vi "lisa_functional.vi"() -> ()   [LabVIEW 2019]
doc: "The classic \"Hello World\" example."
uses:
  <vilib>/Enthought/Python Integration Toolkit/api/Console Visibility.ctl
  <vilib>/Analysis/Matrix/Datatypes/ComplexMatrix.ctl
  <vilib>/Enthought/Python Integration Toolkit/api/Unpack String.vi
  <vilib>/Enthought/Python Integration Toolkit/Python Integration Toolkit.lvlib
  <vilib>/Analysis/Matrix/NI_Matrix.lvlib
panel:
  in  "Mode Coefficients (Cnm)":T1
  in  "beam params. 4":cdb
  in  "b(t) 2":dbl
  in  "Scattering Matrix 2":T1
  in  "Static offsets 2":dbl
  in  "Magnification 2":dbl
  in  "a(t) 2":dbl
  in  "Arm Length 2-3 [m]":dbl
  in  "Arm Length 1-3 [m]":dbl
  in  "b(t)5":dbl
  in  "Scattering Matrix 6":T1
  in  "Static offsets 6":dbl
  in  "Magnification 6":dbl
  in  "a(t)5":dbl
  in  "Arm Length 1-2 [m]":dbl
  in  "b(t)5":dbl
  in  "Scattering Matrix 5":T1
  in  "Static offsets 5":dbl
  in  "Magnification 5":dbl
  in  "a(t)5":dbl
  in  "b(t) 4":dbl
  in  "Scattering Matrix 4":T1
  in  "Static offsets 4":dbl
  in  "Magnification 4":dbl
  in  "a(t) 4":dbl
  in  "C n,m 3":T1
  in  "beam params. 3":cdb
  in  "C n,m 2":T1
  in  "beam params. 2":cdb
  in  "b(t) 3":dbl
  in  "Scattering Matrix 3":T1
  in  "Static offsets 3":dbl
  in  "Magnification 3":dbl
  in  "a(t) 3":dbl
  in  "b(t)":dbl
  in  "Scattering Matrix":T1
  in  "Static offsets":dbl
  in  "Magnification":dbl
  in  "a(t)":dbl
  in  "Mode Coefficients (Cnm)":T1
  in  "beam params.":cdb
  in  "Display Python console?":T2=enum."Hide Console"
  in  "Your name":string="LabVIEW Champion"
  out "Response from Python":string
  # "LISA Optical Metrology Functional Panel"
  # "S/C 1"
  # "S/C 3"
  # "MOSA 3(a)"
  # "MOSA 1(a)"
  # "TM 1(a)"
  # "MOSA 1(b)"
  # "Dynamic\nAng. Offsets"
  # "Dynamic\nAng. Offsets"
  # "TM 1(b)"
  # "MOSA 3(b)"
  # "TM 3(a)"
  # "TM 3(b)"
  # "Laser 1(a)"
  # "Backlink"
  # "Dynamic\nAng. Offsets"
  # "Laser 3"
  # "Dynamic\nAng. Offsets"
  # "TS 1(a)"
  # "TS 1(b)"
  # "TS 3(b)"
  # "PD 1(b)"
  # "PD 1(a)"
  # "TM PD\n1(a)"
  # "OB 1(a)"
  # "PRDS"
  # "OB 1(b)"
  # "TS 3(a)"
  # "PRDS"
  # "TM Im\n1(a)"
  # "Ref Im\n1(a)"
  # "Imaging 1(b)"
  # "Imaging 1(a)"
  # "Laser 1(b)"
  # "RX CLIP 1(b)"
  # "RX CLIP 1(a)"
  # "OB 3(a)"
  # "OB 3(b)"
  # "TX CLIP"
  # "RX CLIP"
  # "TX CLIP 1(a)"
  # "PM(tx/rx) 1(b)"
  # "PM(tx/rx) 1(a)"
  # "TX CLIP 1(b)"
  # "S/C 2"
  # "TM 2(a)"
  # "MOSA 2(a)"
  # "MOSA 2(b)"
  # "TS 2(a)"
  # "TM 2(b)"
  # "Dynamic\nAng. Offsets"
  # "Dynamic\nAng. Offsets"
  # "TS 2(b)"
  # "Laser 2"
  # "OB 2(a)"
  # "OB 2(a)"
  # "TX CLIP"
  # "TX CLIP"
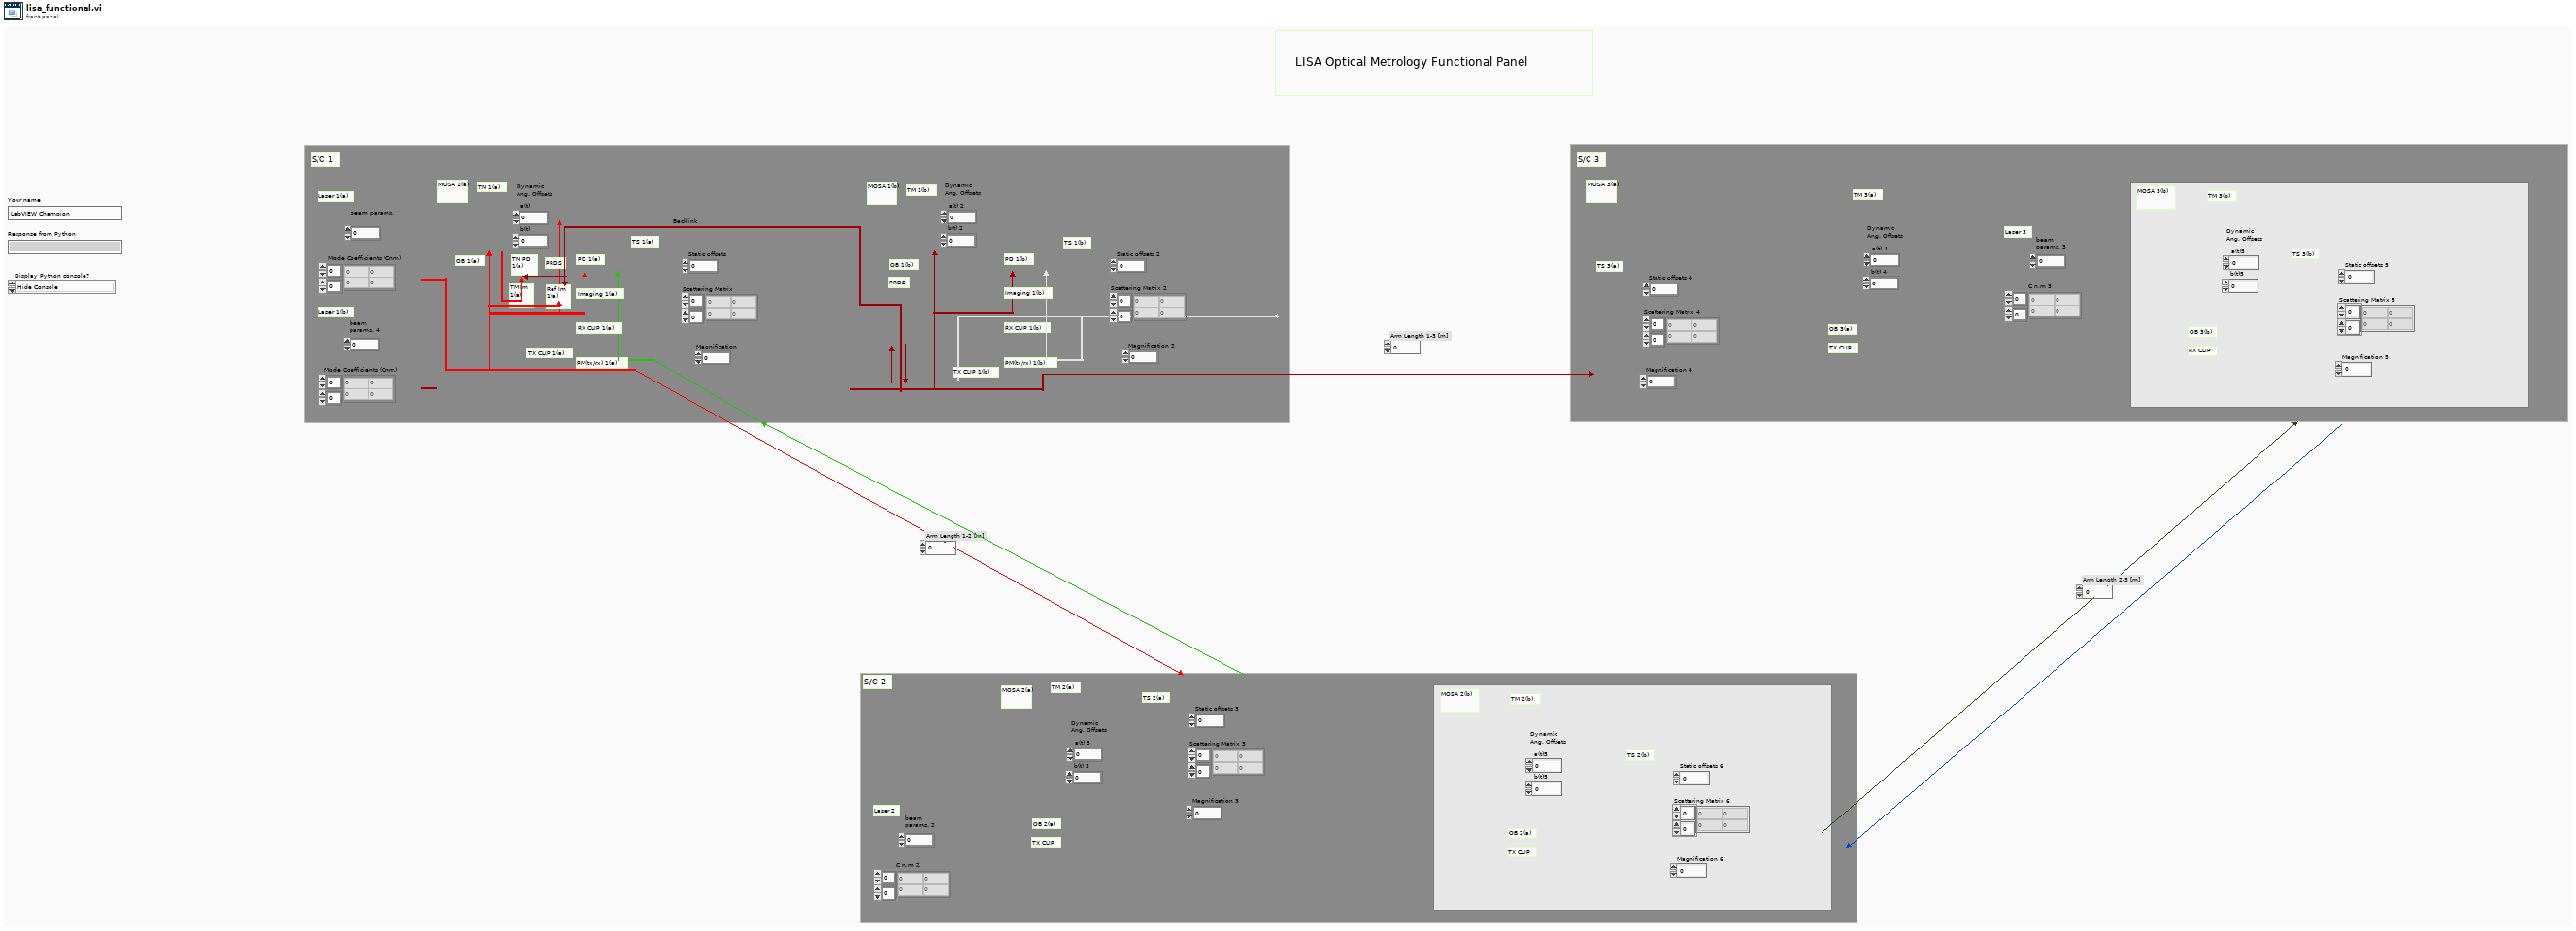
[diagram p1: front panel]
types:
  T1 = typedef "NI_Matrix.lvlib/ComplexMatrix.ctl" = cdb[][]
  T2 = typedef "Python Integration Toolkit.lvlib/Console Visibility.ctl" = enum16{"Show Console", "Show Console While Running", "Hide Console"}
  T3 = typedef "Python Integration Toolkit.lvlib/Session ID.ctl" = u64
  T4 = typedef "Python Integration Toolkit.lvlib/Python Objects.ctl" = variant
  T5 = cluster{"beam params.":cdb, "Mode Coefficients (Cnm)":T1}
  T6 = cluster{cluster{"beam params.":cdb, "Mode Coefficients (Cnm)":T1}, "Scattering Matrix":T1}
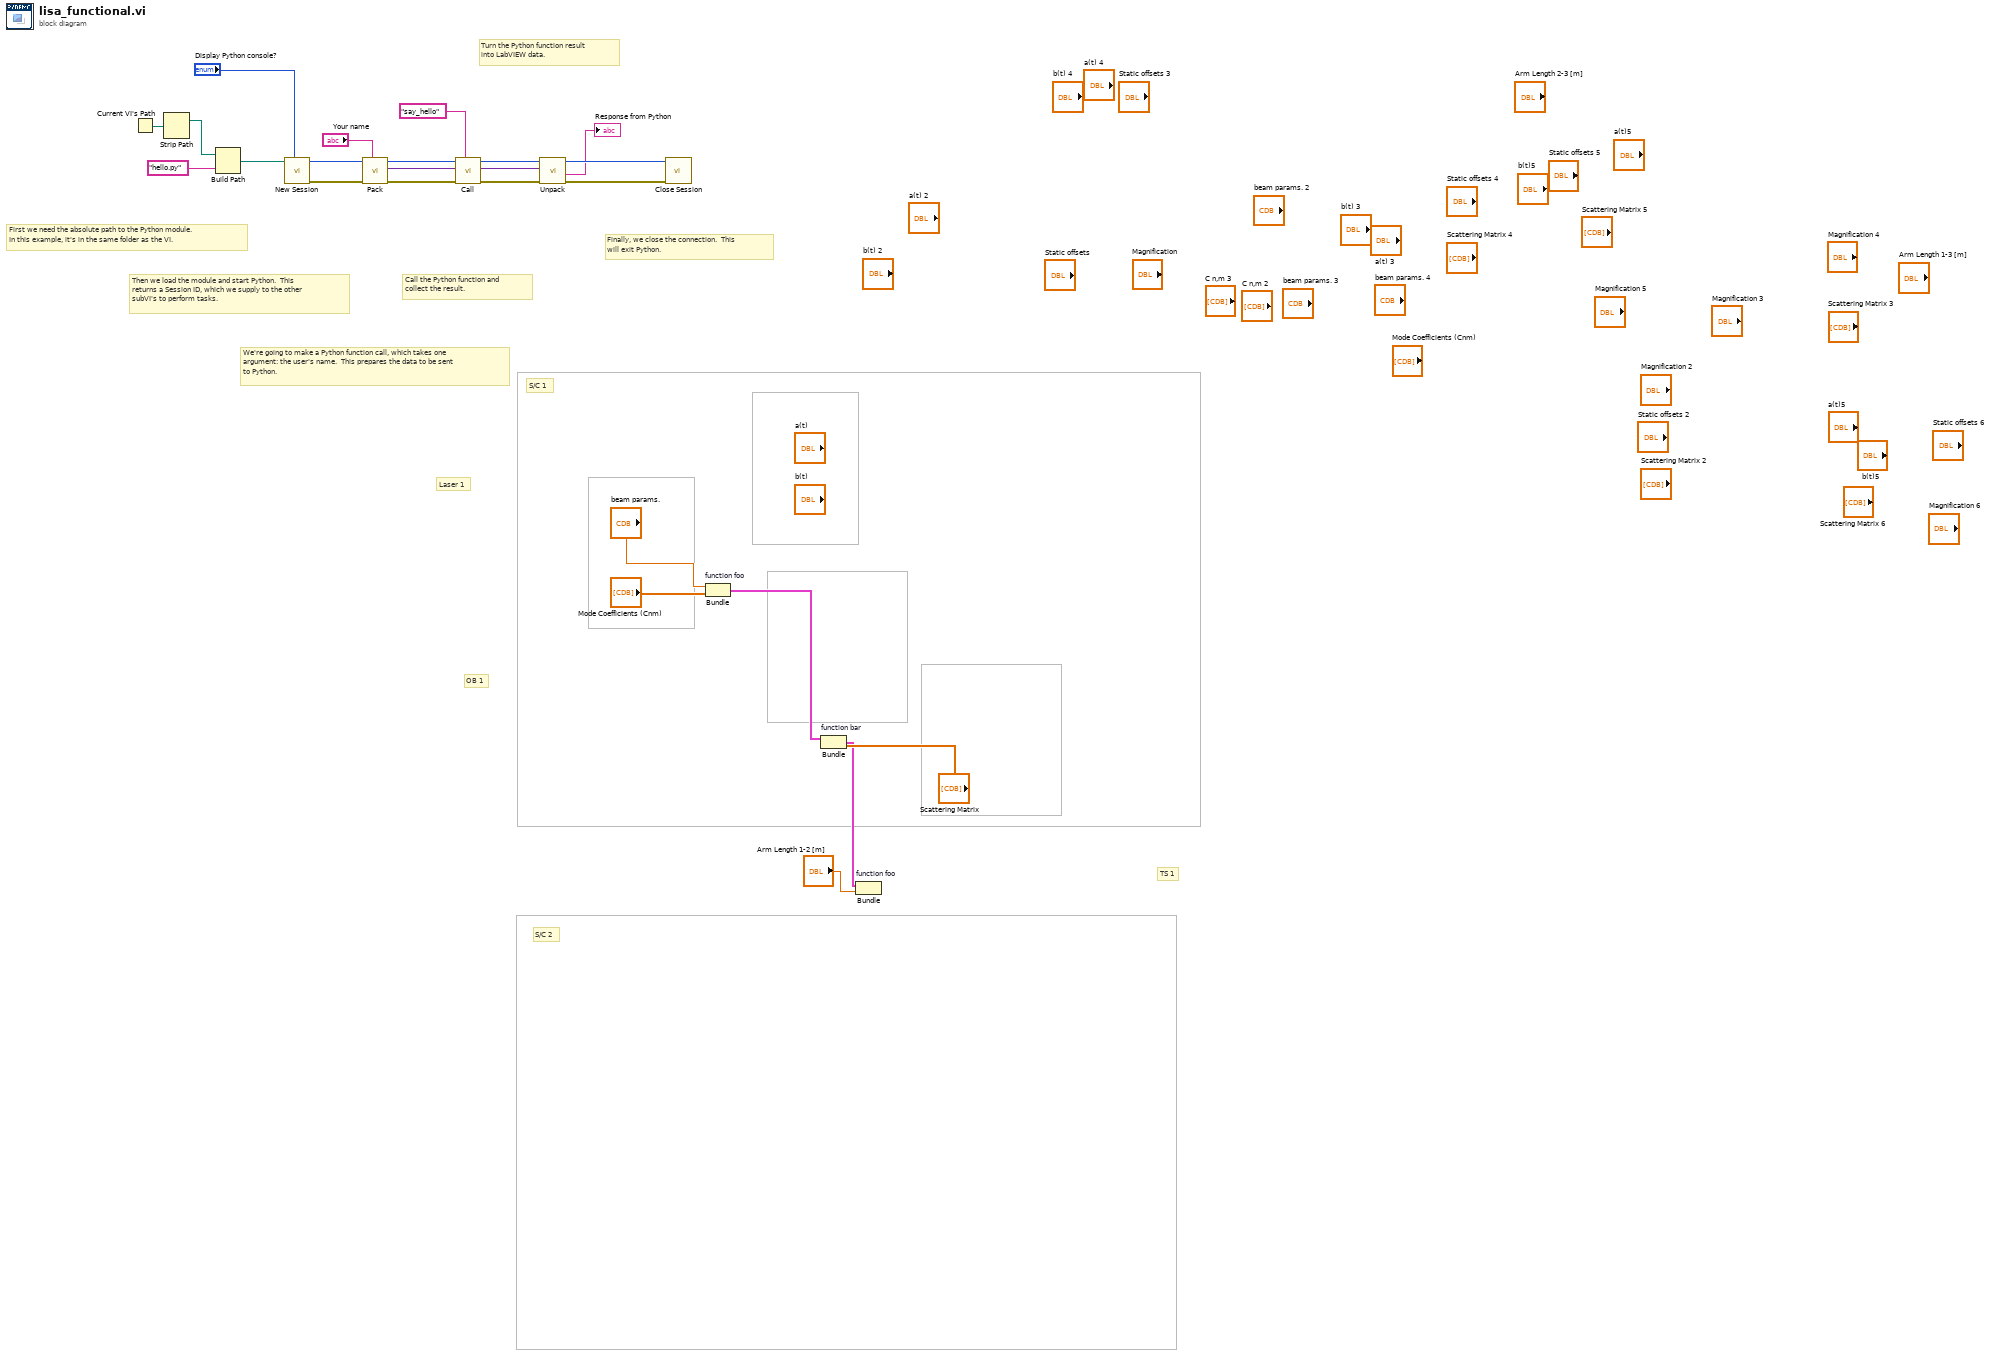
[diagram p0: block diagram]
diagram:
  # "TS 1"
  # "S/C 2"
  # "OB 1"
  # "S/C 1"
  # "Laser 1"
  # "Finally, we close the connection.  This\nwill exit Python."
  # "Turn the Python function result\ninto LabVIEW data."
  # "Call the Python function and\ncollect the result."
  # "We're going to make a Python function call, which takes one\nargument: the user's name.  This prepares the data to be sent\nto Python."
  # "Then we load the module and start Python.  This\nreturns a Session ID, which we supply to the other\nsubVI's to perform tasks."
  # "First we need the absolute path to the Python module.\nIn this example, it's in the same folder as the VI."
  n1 = Current VI's Path() -> (path=w24:path)
  n2 = Strip Path(path=w24) -> (stripped path=w23:path)  [unwired: 1 out]
  n3 = Build Path(base path=w23, name or relative path="hello.py") -> (appended path=w21:path)
  n4 = call <vilib>:"New Session.vi"("Console Visibility"="Display Python console?", "Path to Python Module (.py File)"=w21) -> ("error out"=w13:errorcluster, "Session ID out"=w14:T3)  [unwired: 8 in]
  n5 = call <vilib>:"Pack.vi"("Argument"="Your name", "error in (no error)"=w13, "Session ID"=w14) -> ("error out"=w11:errorcluster, "Python Object References Out"=w8:T4, "Session ID out"=w12:T3)  [unwired: 6 in]
  n6 = call <vilib>:"Call.vi"("Function or Method Name"="say_hello", "error in (no error)"=w11, "Python Object References In"=w8, "Session ID"=w12) -> ("error out"=w19:errorcluster, "Python Object References Out"=w16:T4, "Session ID out"=w20:T3)  [unwired: 5 in]
  n7 = call-poly <vilib>:"Unpack.vi"("error in (no error)"=w19, "Python Object References In"=w16, "Session ID"=w20) -> ("error out"=w17:errorcluster, "Value"=→"Response from Python":string, "Session ID out"=w18:T3)  [unwired: 5 in, 1 out]
  n8 = call <vilib>:"Close Session.vi"("error in (no error)"=w17, "Session ID"=w18) -> ()  [unwired: 9 in, 1 out]
  n9 = Bundle "function foo"("beam params."="beam params.", "Mode Coefficients (Cnm)"="Mode Coefficients (Cnm)") -> (w4:T5)  [unwired: 1 in]
  n10 = Bundle "function bar"(w4, "Scattering Matrix"="Scattering Matrix") -> (w2:T6)  [unwired: 1 in]
  n11 = Bundle "function foo"(w2, "Arm Length 1-2 [m]"="Arm Length 1-2 [m]") -> ()  [unwired: 1 in, 1 out]
